vi "Subvi_Online_For_Offline_Analysis_For_Checking_LDAMatrix_SWLDA.vi"(0 "rate":dbl=500.0 caption="Rate" format="%0.2f", 1 "samples per channel":i32=25, 2 "DIscard Channel Info":i32[](array[numeric]), 5 "Brain_data_source":dbl[][](array[numeric]) caption="EEG_Raw_Data" format="%0.3f", 7 "Target_Flash_Order":i64[][](array[numeric]), 8 "Value":T1, 10 "Weight":dbl[](array[numeric]), 11 "Path":path, 14 "Number":string, 16 "Matrix":T1, 17 "Channel selection":bool[](array[boolean])) -> (13 "LDA_Parameter":dbl[][](array[numeric]), 15 "EPR_발생_total":i16[](array[numeric]), 20 "output-0~8":i32, 22 "ERP_Parameters":dbl[][](array[numeric]), 26 "SWLDA":dbl[](array[numeric]))   [LabVIEW 2014]
uses:
  <vilib>/Analysis/Matrix/Datatypes/RealMatrix.ctl
  <vilib>/Analysis/3filter.llb/Filter Passband Type.ctl
  <vilib>/Analysis/baseanly.llb/Mean (DBL).vi
  <vilib>/Analysis/3filter.llb/Butterworth Filter (DBL).vi
  <vilib>/Analysis/Matrix/Numeric/Conversions/Array To Matrix - RA.vi
  <vilib>/Analysis/Matrix/Numeric/Multiply/Multiply - RM,RM.vi
  <vilib>/Analysis/Matrix/Numeric/Subtract/Subtract - RM,RM.vi
  <vilib>/Analysis/Matrix/Numeric/Conversions/Matrix To Array - RM.vi
  <vilib>/Analysis/NI_AALBase.lvlib
  <vilib>/Analysis/Matrix/NI_Matrix.lvlib
  <vilib>/Utility/file.llb/Read From Spreadsheet File (DBL).vi
  <vilib>/Analysis/Matrix/Numeric/Conversions/Array To Matrix - RA2.vi
panel:
  out "element":i32
  out "A - B":T1
  in  "LDA":path=path "C:/Users/Administrator/Desktop/공공복지안전사업연구-노수진/파일럿20130902/LDA_Matrix_Value.xls"
  out "#channel":i32
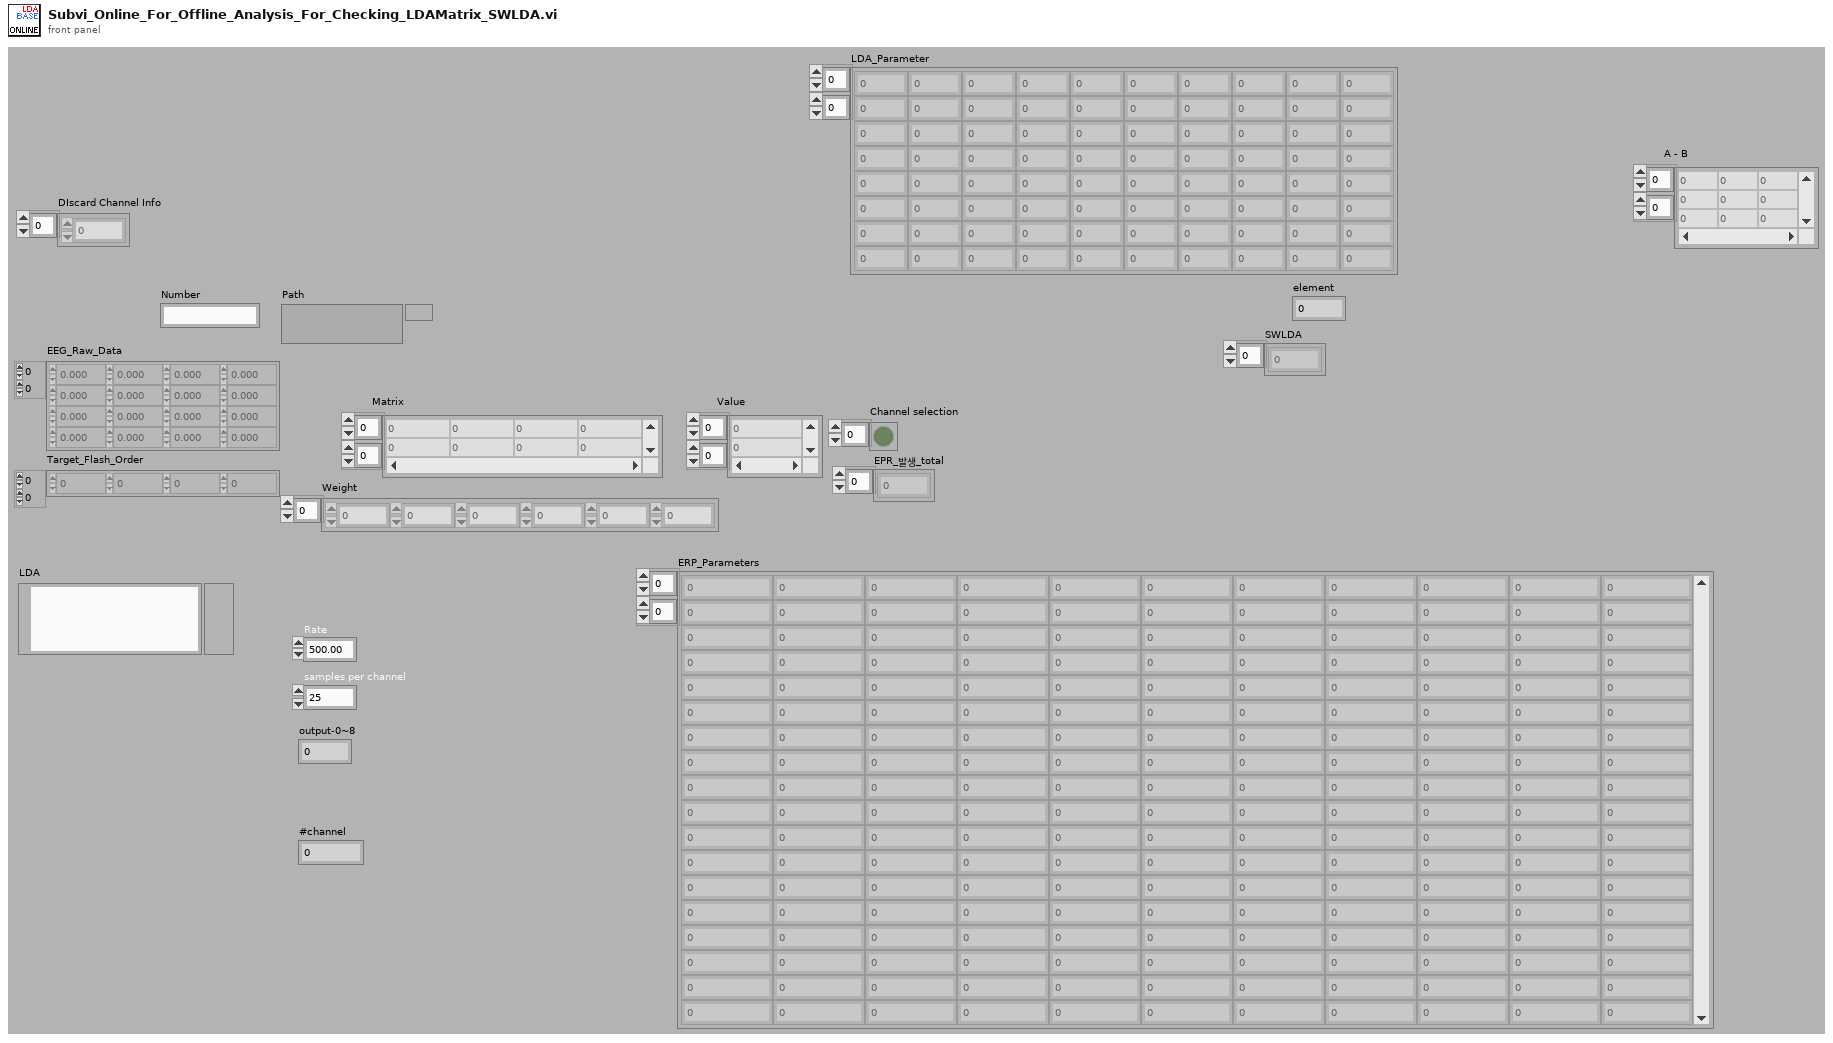
[diagram p1: front panel]
types:
  T1 = typedef "NI_Matrix.lvlib/RealMatrix.ctl" = dbl[][]
  T2 = typedef "NI_AALBase.lvlib/Filter Passband Type.ctl" = enum32{"Lowpass", "Highpass", "Bandpass", "Bandstop"}
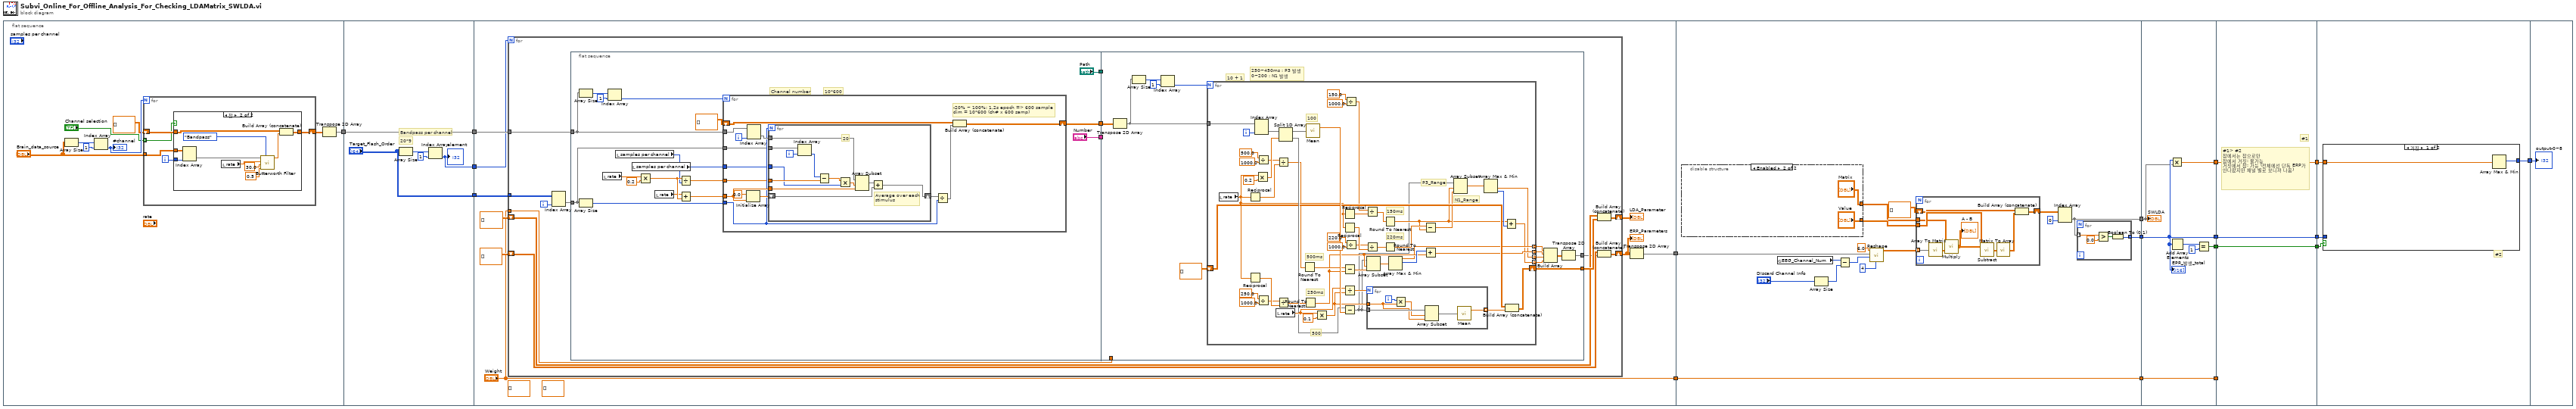
[diagram p0: block diagram]
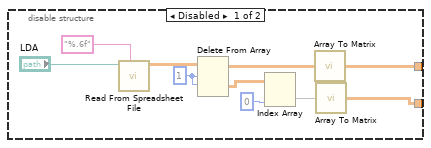
[diagram p3: hidden frame]
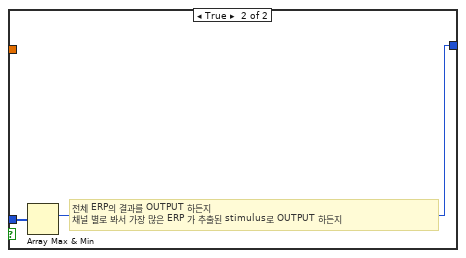
[diagram p4: hidden frame]
diagram:
  n1 = flat-sequence {
    tunnel: [w22] -> w17
    tunnel: [w46] -> w16
    tunnel: ["Target_Flash_Order"] -> w15
    tunnel: w17 -> [w46]
    tunnel: [w43] -> w14
    tunnel: w16 -> [w55]
    tunnel: w15 -> [w54]
    tunnel: w14 -> [w53]
    tunnel: [w47] -> w13
    tunnel: ["Weight"] -> w8
    tunnel: w13 -> [w189]
    tunnel: [w197] -> w12
    tunnel: w8 -> [w195]
    tunnel: [w195] -> w7
    tunnel: [w193] -> w5
    tunnel: w12 -> [w227]
    tunnel: [w229] -> w11
    tunnel: w7 -> [w228]
    tunnel: [w228] -> w6
    tunnel: w5 -> [w225]
    tunnel: [w227] -> w4
    tunnel: [w226] -> w2
    tunnel: w11 -> [w234]
    tunnel: [w234] -> w10
    tunnel: w6 -> [_]
    tunnel: w4 -> [w233]
    tunnel: [w233] -> w3
    tunnel: w2 -> [w232]
    tunnel: [w232] -> w1
    tunnel: [w237] -> w9
    tunnel: w10 -> [w238]
    tunnel: w3 -> [w236]
    tunnel: w1 -> [w235]
    tunnel: w9 -> [w243]
    frame #0 {
      n2 = Array Size(array="Brain_data_source") -> (size(s)=w23:i32[])
      n3 = Index Array(array=w23, index=1) -> (element=w25:i32)
      "#channel" <- w25
      n4 = for {
        N: w25 -> [_]
        tunnel: "Brain_data_source" -> [w30]
        shift-right: [w27] -> w19
        shift-left: dbl[][] [] ("Filtered X") -> [w28]
        tunnel: "Channel selection" -> [w26] mode=indexing
        i -> [w29]
        n5 = case shown="참" w26 {
          tunnel: w30 -> [_ w41]
          tunnel: w29 -> [_ w40]
          tunnel: w28 -> [w31 w34]
          tunnel: [w31 w33] -> w27
          frame False {
          }
          frame True {
            n6 = Index Array(array=w41, index (col)=w40) -> (element=w39:dbl[])  [unwired: 1 in]
            n7 = local read "rate"() -> (w35:dbl)
            n8 = call-poly <vilib>:"Butterworth Filter.vi"("filter type"=Filter_Passband_Type."Bandpass", "low cutoff freq: fl"=0.5, "high cutoff freq: fh"=30.0, "sampling freq: fs"=w35, "X"=w39) -> ("Filtered X"=w32:dbl[])  [unwired: 3 in, 1 out]
            n9 = Build Array (concatenate)(w34, w32) -> (w33:dbl[][])
          }
        }
      }
      n10 = Transpose 2D Array(2D array=w19) -> (transposed array=w22:dbl[][])
    }
    frame #1 {
      # "Bandpass per channel"
      # "20*9"
      n11 = Array Size(array="Target_Flash_Order") -> (size(s)=w45:i32[])
      n12 = Index Array(array=w45, index=1 ("인덱스")) -> (element=w43:i32)
      "element" <- w43
    }
    frame #2 {
      (unwired) dbl[][] []
      (unwired) dbl[][] []
      n13 = for {
        N: w53 -> [_]
        tunnel: w55 -> [w68]
        tunnel: w54 -> [w67]
        shift-right: [w65] -> w51
        shift-left: dbl[][] [] -> [w64]
        shift-right: [w59] -> w49
        shift-left: dbl[][] [] -> [w58]
        tunnel: "Weight" -> [w57]
        i -> [w63]
        n14 = Index Array(array=w67, index (col)=w63) -> (element=w66:i64[])  [unwired: 1 in]
        n15 = flat-sequence {
          tunnel: w68 -> [w74]
          tunnel: w66 -> [w73]
          tunnel: [w72] -> w69
          tunnel: ["Path"] -> w62
          tunnel: ["Number"] -> w61
          tunnel: w69 -> [w124]
          tunnel: [w116] -> w56
          tunnel: w62 -> [_]
          tunnel: w61 -> [_]
          tunnel: [w122] -> w60
          tunnel: w57 -> [_]
          frame #0 {
            # "10*600"
            # "Channel number"
            n16 = Array Size(array=w74) -> (size(s)=w77:i32[])
            n17 = Array Size(array=w73) -> (size(s)=w76:i32)
            n18 = local read "rate"() -> (w83:dbl)
            n19 = Index Array(array=w77, index=1) -> (element=w79:i32)
            n20 = local read "samples per channel"() -> (w81:i32)
            n21 = local read "samples per channel"() -> (w80:i32)
            n22 = Multiply(x=w83, y=0.2) -> (x*y=w87:dbl)
            n23 = local read "rate"() -> (w85:dbl)
            n24 = Divide(x=w87, y=w81) -> (x/y=w84:dbl)
            n25 = Add(x=w85, y=w87) -> (x+y=w86:dbl)
            n26 = for {
              N: w79 -> [_]
              tunnel: w80 -> [w88]
              tunnel: w86 -> [w99]
              shift-right: [w92] -> w72
              shift-left: dbl[][] [] -> [w94]
              tunnel: w76 -> [w93]
              tunnel: w74 -> [w91]
              tunnel: w73 -> [w90]
              tunnel: w84 -> [w89]
              i -> [w101]
              # "-20% ~ 100%: 1.2s epoch => 600 sample\ndim = 10*600 (ch# x 600 samp)"
              n27 = Initialize Array(0.0 ("element"), w99) -> (w98:dbl[])
              n28 = Index Array(array=w91, index (col)=w101) -> (element=w100:dbl[])  [unwired: 1 in]
              n29 = for {
                N: w93 -> [_]
                tunnel: w100 -> [w113]
                shift-right: [w110] -> w96
                shift-left: w98 -> [w111]
                tunnel: w99 -> [w109]
                tunnel: w90 -> [w107]
                tunnel: w89 -> [w105]
                tunnel: w88 -> [w103]
                i -> [w108]
                # "Average over each\nstimulus"
                # "20"
                n30 = Index Array(array=w107, index=w108) -> (element=w106:i64)
                n31 = Subtract(x=w106, y=w105) -> (x-y=w104:dbl)
                n32 = Multiply(x=w104, y=w103) -> (x*y=w102:dbl)
                n33 = Array Subset(array=w113, index=w102, length=w109) -> (w112:dbl[])
                n34 = Add(x=w112, y=w111) -> (x+y=w110:dbl[])
              }
              n35 = Divide(x=w96, y=w93) -> (x/y=w95:dbl[])
              n36 = Build Array (concatenate)(w94, w95) -> (w92:dbl[][])
            }
          }
          frame #1 {
            # "250~450ms : P3 발생\n0~200 : N1 발생"
            # "10 + 1"
            n37 = Transpose 2D Array(2D array=w124) -> (transposed array=w114:dbl[][])
            n38 = Array Size(array=w114) -> (size(s)=w125:i32[])
            n39 = Index Array(array=w125, index=1) -> (element=w115:i32)
            n40 = for {
              N: w115 -> [_]
              tunnel: w114 -> [w177]
              tunnel: [w130] -> w121 mode=indexing
              tunnel: [w129] -> w120 mode=indexing
              tunnel: [w128] -> w119 mode=indexing
              tunnel: [w127] -> w118 mode=indexing
              shift-right: [w163] -> w122
              shift-left: dbl[][] [] -> [w162]
              i -> [w166]
              # "N1_Range"
              # "P3_Range"
              # "220ms"
              # "150ms"
              # "500ms"
              # "250ms"
              # "500"
              # "100"
              n41 = local read "rate"() -> (w144:dbl)
              n42 = Reciprocal(x=w144) -> (1/x=w159:dbl)
              n43 = Reciprocal(x=w144) -> (1/x=w160:dbl)
              n44 = Index Array(array=w177, index (col)=w166) -> (element=w168:dbl[])  [unwired: 1 in]
              n45 = Multiply(x=w144, y=0.2) -> (x*y=w175:dbl)
              n46 = Divide(x=500.0, y=1000.0) -> (x/y=w155:dbl)
              n47 = Divide(x=250.0, y=1000.0) -> (x/y=w156:dbl)
              n48 = local read "rate"() -> (w171:dbl)
              n49 = Divide(x=w155, y=w159) -> (x/y=w142:dbl)
              n50 = Divide(x=w156, y=w160) -> (x/y=w143:dbl)
              n51 = Split 1D Array(array=w168, index=w175) -> (first subarray=w174:dbl[], second subarray=w165:dbl[])
              n52 = Round To Nearest(number=w142) -> (nearest integer value=w139:dbl)
              n53 = Round To Nearest(number=w143) -> (nearest integer value=w132:dbl)
              n54 = call-poly <vilib>:"Mean.vi"("X"=w174) -> ("mean"=w173:dbl)  [unwired: 1 out]
              n55 = Multiply(x=w171, y=0.1) -> (x*y=w164:dbl)
              n56 = Reciprocal(x=w144) -> (1/x=w158:dbl)
              n57 = Reciprocal(x=w144) -> (1/x=w157:dbl)
              n58 = Subtract(x=w139, y=w132) -> (x-y=w137:dbl)
              n59 = Divide(x=w171, y=w164) -> (x/y=w170:dbl)
              n60 = Subtract(x=w165, y=w173) -> (x-y=w131:dbl[])
              n61 = Divide(x=150.0, y=1000.0) -> (x/y=w154:dbl)
              n62 = Divide(x=220.0, y=1000.0) -> (x/y=w153:dbl)
              n63 = Divide(x=w154, y=w158) -> (x/y=w141:dbl)
              n64 = Divide(x=w153, y=w157) -> (x/y=w140:dbl)
              n65 = Array Subset(array=w131, index=w132, length=w137) -> (w135:dbl[])
              n66 = for {
                N: w170 -> [_]
                tunnel: w131 -> [w182]
                tunnel: [w183] -> w161 mode=indexing
                tunnel: w164 -> [w180]
                i -> [w179]
                n67 = Multiply(x=w179, y=w180) -> (x*y=w181:dbl)
                n68 = Array Subset(array=w182, index=w181, length=w180) -> (w178:dbl[])
                n69 = call-poly <vilib>:"Mean.vi"("X"=w178) -> ("mean"=w183:dbl)  [unwired: 1 out]
              }
              n70 = Round To Nearest(number=w141) -> (nearest integer value=w133:dbl)
              n71 = Round To Nearest(number=w140) -> (nearest integer value=w138:dbl)
              n72 = Array Max & Min(array=w135) -> (max value=w130:dbl, max index (indices)=w169:i32)  [unwired: 2 out]
              n73 = Subtract(x=w138, y=w133) -> (x-y=w136:dbl)
              n74 = Add(x=w169, y=w132) -> (x+y=w129:dbl)
              n75 = Array Subset(array=w131, index=w133, length=w136) -> (w134:dbl[])
              n76 = Array Max & Min(array=w134) -> (min value=w128:dbl, min index (indices)=w167:i32)  [unwired: 2 out]
              n77 = Add(x=w133, y=w167) -> (x+y=w127:dbl)
              n78 = Build Array (concatenate)(w162, w161) -> (w163:dbl[][])
            }
            n79 = Build Array(w121, w120, w119, w118) -> (w117:dbl[][])
            n80 = Transpose 2D Array(2D array=w117) -> (transposed array=w116:dbl[][])
          }
        }
        n81 = Build Array (concatenate)(w58, w60) -> (w59:dbl[][])
        n82 = Build Array (concatenate)(w64, w56) -> (w65:dbl[][])
      }
      "ERP_Parameters" <- w51
      "LDA_Parameter" <- w49
      n83 = Transpose 2D Array(2D array=w51) -> (transposed array=w47:dbl[][])
    }
    frame #3 {
      n84 = disable-structure shown="Enabled" {
        disable-tunnel: [w204 "Matrix"] -> w192
        disable-tunnel: [w203 "Value"] -> w196
        frame Disabled {
          w206 = 1 ("인덱스 (행)")
          n85 = call-poly <vilib>:"Read From Spreadsheet File.vi"("format (%.3f)"="%.6f", "file path (dialog if empty)"="LDA") -> ("all rows"=w200:dbl[][])  [unwired: 5 in, 4 out]
          n86 = Delete From Array(array=w200, length=w206, index (row)=w206) -> (deleted portion=w209:dbl[][], array with subset deleted=w208:dbl[][])  [unwired: 1 in]
          n87 = Index Array(array=w209, index (col)=0 ("인덱스")) -> (element=w207:dbl[])  [unwired: 1 in]
          n88 = call-poly <vilib>:"Array To Matrix.vi"("Real 2D Array"=w208) -> ("Real Matrix"=w204:T1)
          n89 = call-poly <vilib>:"Array To Matrix.vi"("Real 1D Array"=w207) -> ("Real Matrix (Column Vector)"=w203:T1)
        }
        frame Enabled {
        }
      }
      n90 = global read "Control_Panel_정리.vi" "EEG_Channel_Num"() -> (w186:i32)
      n91 = Array Size(array="DIscard Channel Info") -> (size(s)=w184:i32)
      n92 = Subtract(x=w186, y=w184) -> (x-y=w187:i32)
      n93 = call "Reshape.vi"("Numeric"=4, "EEG_Channel_Num"=w187, "all rows"=w189, "Numeric 2"=6.0) -> ("Array"=w188:dbl[][])  [unwired: 7 in]
      n94 = for {
        tunnel: w192 -> [w216]
        tunnel: w196 -> [w223]
        shift-right: [w221] -> w198
        shift-left: dbl[][] [] -> [w220]
        tunnel: w188 -> [w219] mode=indexing
        n95 = call-poly <vilib>:"Array To Matrix.vi"("Real 1D Array"=w219) -> ("Real Matrix (Column Vector)"=w217:T1)
        n96 = call-poly <vilib>:"Multiply.vi"("Real Matrix B"=w217, "Real Matrix A"=w216) -> ("A * B"=w218:T1)
        "A - B" <- w218
        n97 = call-poly <vilib>:"Subtract.vi"("Real Matrix B"=w223, "Real Matrix A"=w218) -> ("A - B"=w224:T1)
        n98 = call-poly <vilib>:"Matrix To Array.vi"("Real Matrix"=w224) -> ("Real 2D Array"=w222:dbl[][])
        n99 = Build Array (concatenate)(w220, w222) -> (w221:dbl[][])
      }
      n100 = Index Array(array=w198, index (col)=0 ("비활성화된 인덱스 (열)")) -> (element=w193:dbl[])  [unwired: 1 in]
      n101 = for {
        tunnel: w193 -> [w215] mode=indexing
        tunnel: [w214] -> w197 mode=indexing
        n102 = Greater?(x=w215, y=0.0) -> (0:w212:bool)
        n103 = Boolean To (0,1)(Boolean=w212) -> (0, 1=w214:i16)
      }
    }
    frame #4 {
      n104 = Multiply(x=w227, y=w225) -> (x*y=w226:dbl[])
      n105 = Add Array Elements(numeric array=w227) -> (sum=w231:i16)
      n106 = Equal?(x=w231, y=i16 1) -> (x = y?=w229:bool)
      "EPR_발생_total" <- w227
      "SWLDA" <- w225
    }
    frame #5 {
      # "#1> #2\n참에서는 참으로만\n참에서 거짓: 불가능\n거짓에서 참: 가능 (전체에선 단독 ERP가 안나왔지만 채널 별로 보니까 나옴)"
      # "#1"
    }
    frame #6 {
      # "#2"
      n107 = case shown="거짓" w238 {
        tunnel: [w240 w242] -> w237
        tunnel: w236 -> [_ w241]
        tunnel: w235 -> [w239 _]
        frame False {
          n108 = Array Max & Min(array=w239) -> (max index (indices)=w240:i32)  [unwired: 3 out]
        }
        frame True {
          # "전체 ERP의 결과를 OUTPUT 하든지\n채널 별로 봐서 가장 많은 ERP 가 추출된 stimulus로 OUTPUT 하든지"
          n109 = Array Max & Min(array=w241) -> (max index (indices)=w242:i32)  [unwired: 3 out]
        }
      }
    }
    frame #7 {
      "output-0~8" <- w243
    }
  }
